vi "toml_api_list_keys.vi"(7 "resolved path":path, 8 "error in (no error)":errorcluster, 10 "section":string, 11 "vi in":refnum<vi>) -> (0 "error out":errorcluster, 1 "keys":string[](array[string]), 2 "section exists":bool, 3 "vi out":refnum<vi>)   [LabVIEW 2017]
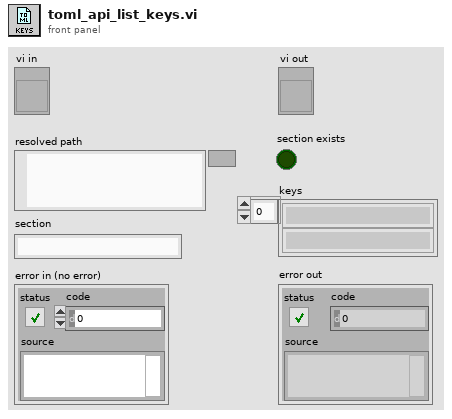
[diagram p1: front panel]
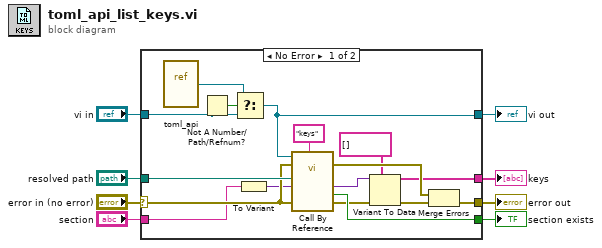
[diagram p0: block diagram]
diagram:
  n1 = case shown="No Error" "error in (no error)" {
    selector: "error in (no error)" -> [w17 w27]
    tunnel: [w25 _] -> w8
    tunnel: "resolved path" -> [w23 _]
    tunnel: [w19 w27] -> w6
    tunnel: "vi in" -> [w16 w26]
    tunnel: [w15 w26] -> w3
    tunnel: [w11 _] -> w2
    tunnel: "section" -> [w10 _]
    frame No Error {
      n2 = vi-ref "toml_api.vi"() -> (w22:refnum<vi>)
      n3 = Not A Number/Path/Refnum?(number/path/refnum=w16) -> (NaN/Path/Refnum?=w21:bool)
      n4 = Select(t=w22, s=w21, f=w16) -> (s? t:f=w15:refnum<vi>)
      n5 = To Variant(anything=w10) -> (Variant=w9:variant)
      n6 = call-by-ref "?"(reference=w15, error in=w17, "cmd"="keys", 8:"error in (no error)"=w17, "data in"=w9, "path in"=w23) -> (error out=w18:errorcluster, 0:"error out"=w24:errorcluster, "return"=w25:bool, "data out"=w13:variant)  [unwired: 4 in, 2 out]
      n7 = Variant To Data(error in=w24, type=string[] [], Variant=w13) -> (data=w11:string[], error out=w14:errorcluster)
      n8 = Merge Errors(w18, w14) -> (w19:errorcluster)
    }
    frame Error {
    }
  }
  "section exists" <- w8
  "error out" <- w6
  "vi out" <- w3
  "keys" <- w2
